vi "AlliGator Settings Event Refnum.vi"(1 "AlliGator Settings Event":T1, 3 "Error In":errorcluster) -> (7 "AlliGator Settings Event Refnum":refnum<user-event>, 9 "Error Out":errorcluster)   [LabVIEW 2021, in "AlliGator Settings.lvlib"]
doc: "Sends user event to the Settings window."
uses:
  AlliGator Settings.lvlib
  AlliGator Settings Event.ctl
  AlliGator Settings Window Messages.ctl
panel:
  # "see the AlliGator License on the block diagram (Ctrl+E or Window:Show Block Diagram)"
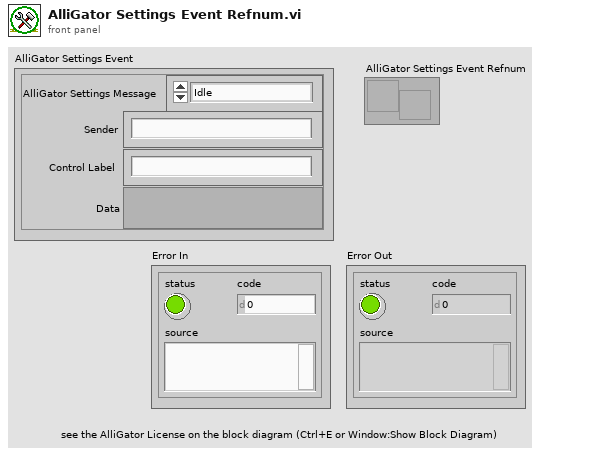
[diagram p1: front panel]
types:
  T1 = typedef "AlliGator Settings.lvlib/AlliGator Settings Event.ctl" = cluster{"AlliGator Settings Message":T2, "Sender":string, "Control Label":string, "Data":variant}
  T2 = typedef "AlliGator Settings.lvlib/AlliGator Settings Window Messages.ctl" = enum16{"Idle", "Subscribe", "Unsubscribe", "Refresh Parameter", "Refresh All Parameters", "Quit"}
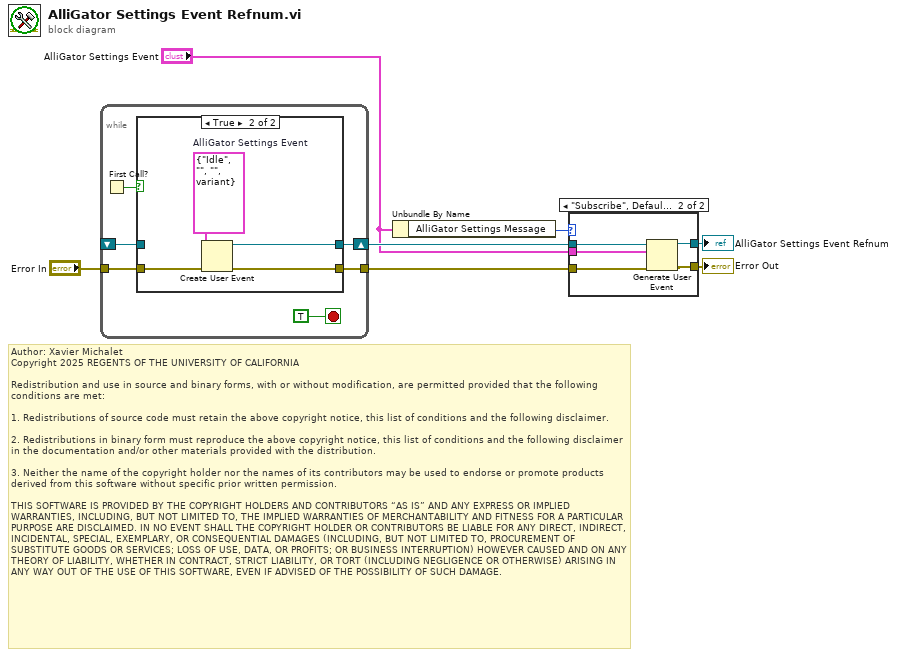
[diagram p0: block diagram]
diagram:
  # "Author: Xavier Michalet\nCopyright 2025 REGENTS OF THE UNIVERSITY OF CALIFORNIA\n\nRedistribution and use in source and binary forms, with or without modification, are permitted provided that the following conditions are met:\n\n1. Redistributions of source code must retain the above copyright notice, this list of conditions and the following disclaimer.\n\n2. Redistributions in binary form must reproduce the above copyright notice, this list of conditions and the following disclaimer in the documentation and/or other materials provided with the distribution.\n\n3. Neither the name of the copyright holder nor the names of its contributors may be used to endorse or promote products derived from this software without specific prior written permission.\n\nTHIS SOFTWARE IS PROVIDED BY THE COPYRIGHT HOLDERS AND CONTRIBUTORS “AS IS” AND ANY EXPRESS OR IMPLIED WARRANTIES, INCLUDING, BUT NOT LIMITED TO, THE IMPLIED WARRANTIES OF MERCHANTABILITY AND FITNESS FOR A PARTICULAR PURPOSE ARE DISCLAIMED. IN NO EVENT SHALL THE COPYRIGHT HOLDER OR CONTRIBUTORS BE LIABLE FOR ANY DIRECT, INDIRECT, INCIDENTAL, SPECIAL, EXEMPLARY, OR CONSEQUENTIAL DAMAGES (INCLUDING, BUT NOT LIMITED TO, PROCUREMENT OF SUBSTITUTE GOODS OR SERVICES; LOSS OF USE, DATA, OR PROFITS; OR BUSINESS INTERRUPTION) HOWEVER CAUSED AND ON ANY THEORY OF LIABILITY, WHETHER IN CONTRACT, STRICT LIABILITY, OR TORT (INCLUDING NEGLIGENCE OR OTHERWISE) ARISING IN ANY WAY OUT OF THE USE OF THIS SOFTWARE, EVEN IF ADVISED OF THE POSSIBILITY OF SUCH DAMAGE."
  n1 = while {
    shift-right: [w11] -> w5
    shift-left: _ -> [w10]
    tunnel: [w9] -> w6
    tunnel: "Error In" -> [w8]
    stop <- TRUE stop-if-true
    n2 = First Call?() -> (First Call?: T/F=w13:bool)
    n3 = case shown="True" w13 {
      tunnel: [w15 w19] -> w11
      tunnel: w10 -> [w15 _]
      tunnel: [w14 w18] -> w9
      tunnel: w8 -> [w14 w17]
      frame False {
      }
      frame True {
        w16 = T1 {"AlliGator Settings Message"=enum."Idle", "Sender"="", "Control Label"="", "Data"=variant}  # AlliGator Settings Event
        n4 = Create User Event(user event datatype=w16, error in=w17) -> (user event=w19:refnum<user-event>, error out=w18:errorcluster)
      }
    }
  }
  n5 = Unbundle By Name("AlliGator Settings Event") -> ("AlliGator Settings Message"=w1:T2)
  n6 = case shown="\"Subscribe\", Default" w1 {
    tunnel: w6 -> [w20 w26]
    tunnel: w5 -> [w21 w25]
    tunnel: [w20 w24] -> w4
    tunnel: "AlliGator Settings Event" -> [_ w23]
    tunnel: [w21 w22] -> w3
    frame "Idle" {
    }
    frame "Subscribe", Default {
      n7 = Generate User Event(user event=w25, event data cluster=w23, error in=w26) -> (user event out=w22:refnum<user-event>, error out=w24:errorcluster)  [unwired: 1 in]
    }
  }
  "Error Out" <- w4
  "AlliGator Settings Event Refnum" <- w3
